vi "Check_Execution_Row.vi"(0 "Execution Row":T1 {"Row Duration (mins)" format="%#.1f"; "Row No" min=0; "Trace Gas Concentration (%)" min=0.0 format="%#.2f"; "Emission Rate (l/min)" format="%#.2f"; "Tunnel Speed" format="%#.2f"; "Start X" format="%#.2f"; "Start Y" format="%#.2f"; "Start Z" format="%#.2f"; "End X" format="%#.2f"; "End Y" format="%#.2f"; "End Z" format="%#.2f"; "Averaging time (min)" min=0.0 format="%#.2f"}, 3 "Synchronization Start No":i32=1 min=1 max=100, 4 "Row Index":i32, 5 "Max Tunnel Speed":dbl format="%.2f") -> (6 "Editted Row":bool, 7 "Execution Row Out":T1 {"Row Duration (mins)" format="%#.1f"; "Row No" min=0; "Trace Gas Concentration (%)" min=0.0 format="%#.2f"; "Emission Rate (l/min)" format="%#.2f"; "Tunnel Speed" format="%#.2f"; "Start X" format="%#.2f"; "Start Y" format="%#.2f"; "Start Z" format="%#.2f"; "End X" format="%#.2f"; "End Y" format="%#.2f"; "End Z" format="%#.2f"; "Averaging time (min)" min=0.0 format="%#.2f"}, 9 "Continue?":bool, 10 "Error Comments":string)   [LabVIEW 2011]
uses:
  Traverse_cluster.ctl
  Spacing.ctl
  Controls/Multi_run_mode.ctl
  Controls/User_Specific_mode.ctl
  Controls/Tunnel_Coordinates.ctl
  ADAM Client/Sub VIs/ADAM Controls/Channel_names.ctl
  Globals/Extra_Commands_Global.vi
  Globals/Constants_global.vi
  Globals/Trav_pos_global.vi
panel:
  out "Traverse line Out":T1 {"Row Duration (mins)" format="%#.1f"; "Row No" min=0; "Trace Gas Concentration (%)" min=0.0 format="%#.2f"; "Emission Rate (l/min)" format="%#.2f"; "Tunnel Speed" format="%#.2f"; "Start X" format="%#.2f"; "Start Y" format="%#.2f"; "Start Z" format="%#.2f"; "End X" format="%#.2f"; "End Y" format="%#.2f"; "End Z" format="%#.2f"; "Averaging time (min)" min=0.0 format="%#.2f"}
  out "Fixed Axis":bool[](array[boolean])
  out "Filenames":string[](array[string])
  out "Current Sync Number":i32
  out "Checks":string[](array[string])
  in  "Edit in Excel":bool
  in  "OK":bool
  # "X           Y            Z"
  # "Start"
  # "End"
  # "X           Y            Z"
  # "Start"
  # "End"
  # "X           Y            Z"
  # "Start"
  # "End"
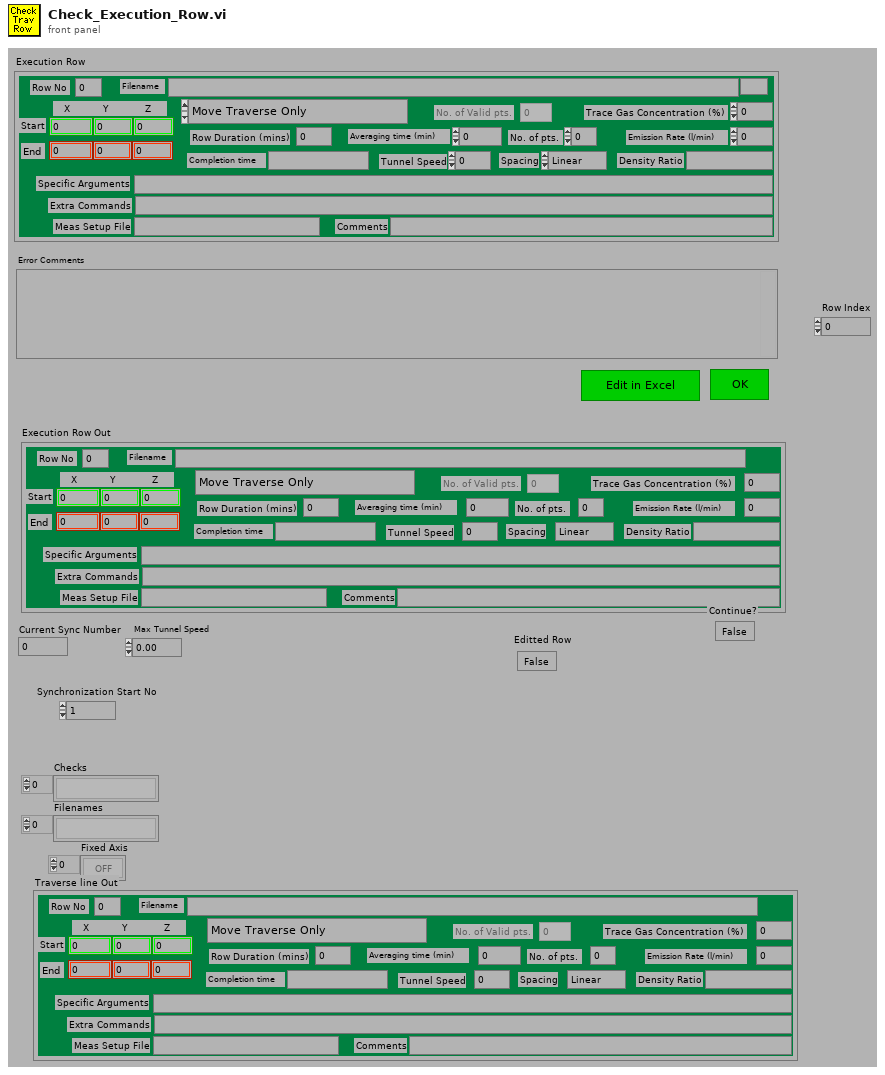
[diagram p1: front panel]
types:
  T1 = typedef "Traverse_cluster.ctl" = cluster{"Start X":dbl, "Start Y":dbl, "Start Z":dbl, "End X":dbl, "End Y":dbl, "End Z":dbl, "No. of pts.":i32, "Spacing":T2, "Filename":path, "Tunnel Speed":dbl, "Averaging time (min)":dbl, "Extra Commands":string, "Specific Arguments":string, "Emission Rate (l/min)":dbl, "Trace Gas Concentration (%)":dbl, "Density Ratio":string, "Comments":string, "Row No":i32, "Row Type Selector":T3, "Completion time":string, "Row Duration (mins)":dbl, "No. of Valid pts.":i32, "Meas Setup File":string}
  T2 = typedef "Spacing.ctl" = enum16{"Linear", "Log", "Gauss", "Specified", "N/A"}
  T3 = typedef "Multi_run_mode.ctl" = enum16{"Move Traverse Only", "Set Tunnel Speed Only", "Set Source Only", "Set Measurement Conditions", "Single Measurement", "Vertical Profile", "Lateral Profile", "Longitudinal Profile", "Explore Volume", "Multi-Axis Profile", "Auto Calibrate", "Meas Fast FID Bkgnd", "Check Beam Power", "Scanning Valve Measurement", "Run VI Named:", "Set ADAM Ch", "Wait (minutes)", "Send Message", "Synchronize With:", "Fall Back to this Row", "Turn Off Row Repeating", "Blank Row", "Traverse 3D Volume"}
  T4 = enum16{"All Channel Names", "Valid Channel Names"}
  T5 = typedef "User_Specific_mode.ctl" = enum16{"Check VI only", "Run VI"}
  T6 = typedef "Tunnel_Coordinates.ctl" = enum16{"Work in Tunnel Coordinates", "Work in Model Coordinates"}
  T7 = enum16{"Zero or one", "One", "Zero or more", "One or more"}
  T8 = typedef "Channel_names.ctl" = enum16{"Active Only", "Active + Off", "All Channels"}
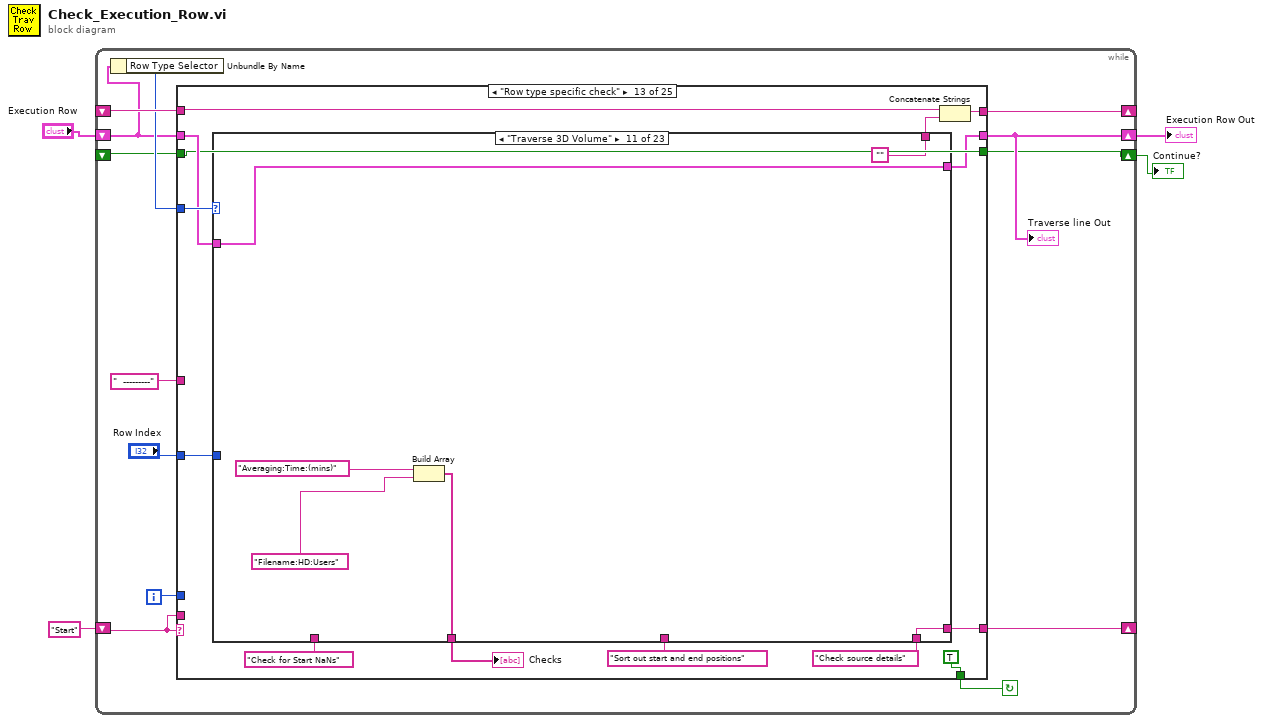
[diagram p0: block diagram]
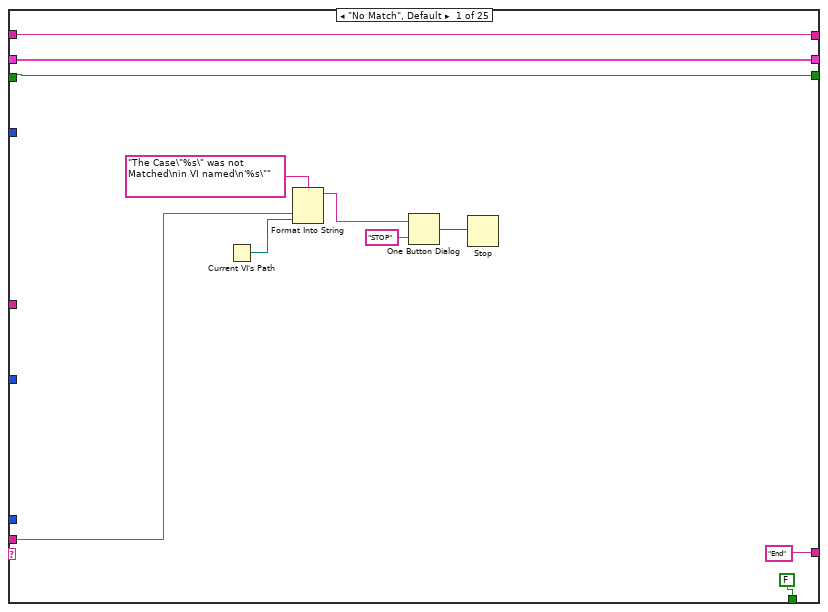
[diagram p2: hidden frame]
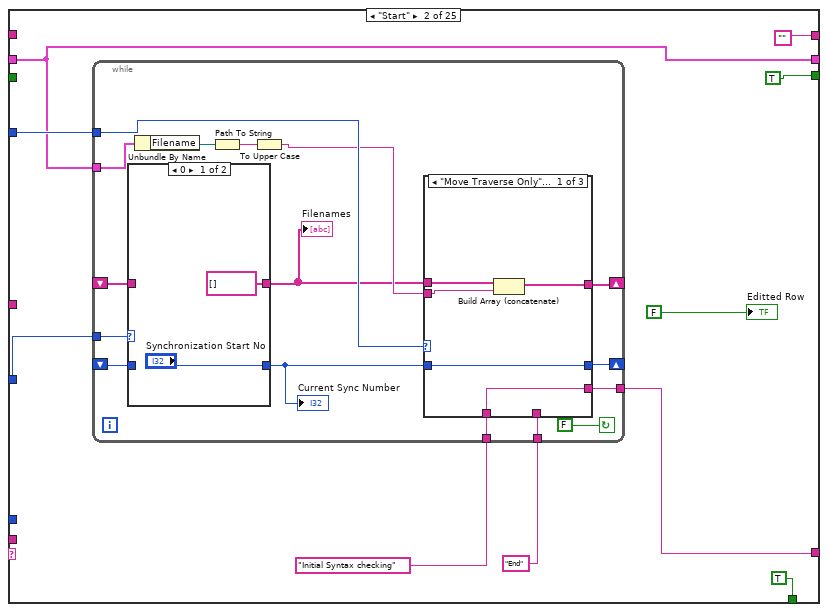
[diagram p3: hidden frame]
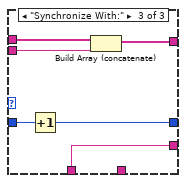
[diagram p6: hidden frame]
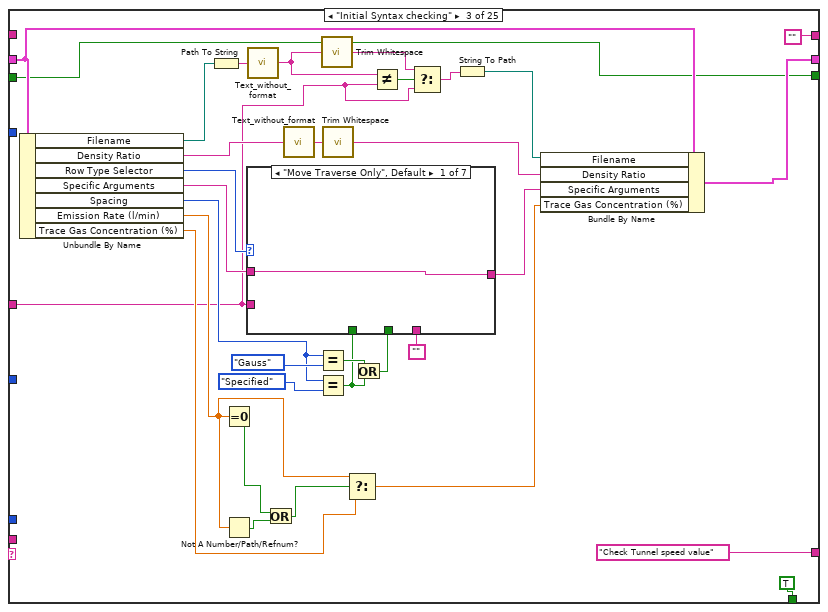
[diagram p7: hidden frame]
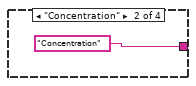
[diagram p9: hidden frame]
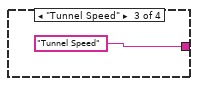
[diagram p10: hidden frame]
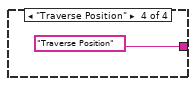
[diagram p11: hidden frame]
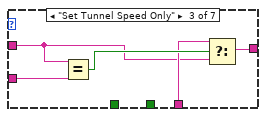
[diagram p12: hidden frame]
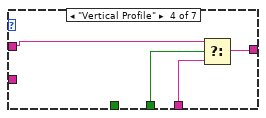
[diagram p13: hidden frame]
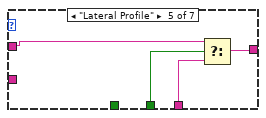
[diagram p14: hidden frame]
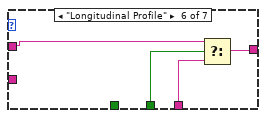
[diagram p15: hidden frame]
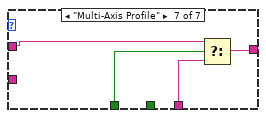
[diagram p16: hidden frame]
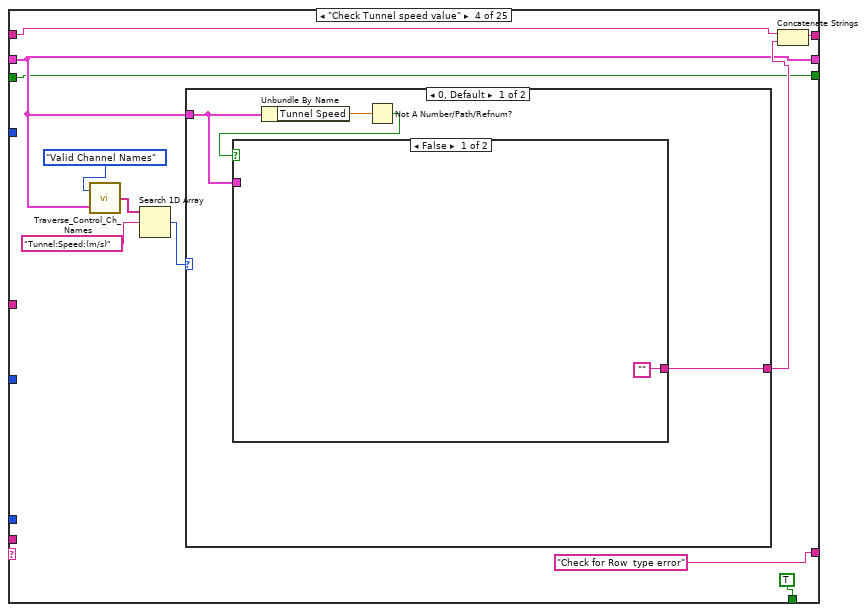
[diagram p17: hidden frame]
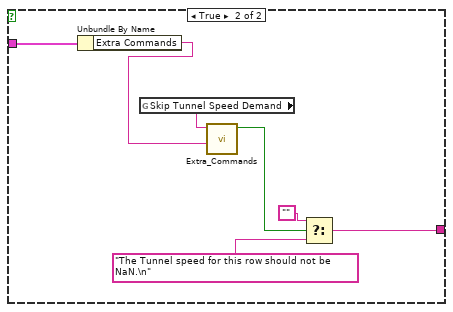
[diagram p18: hidden frame]
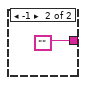
[diagram p19: hidden frame]
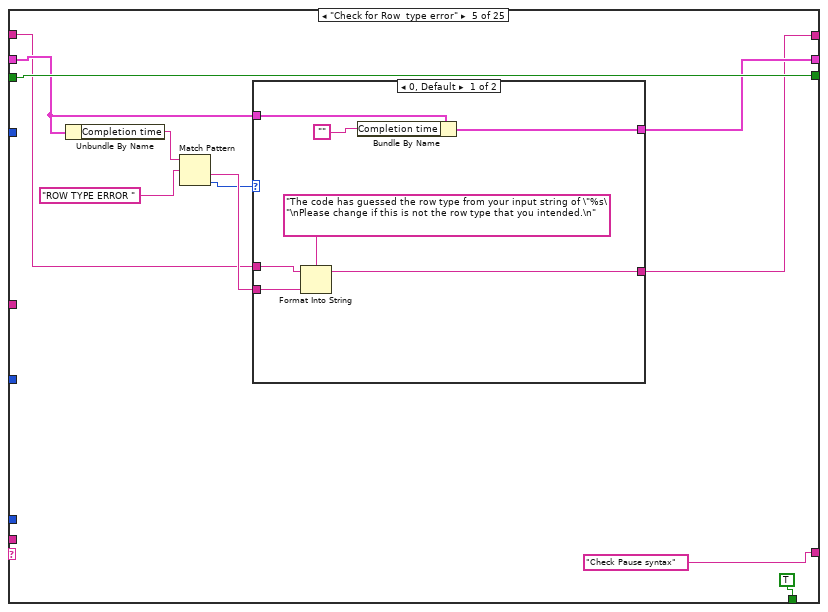
[diagram p20: hidden frame]
diagram:
  n1 = while {
    shift-left: _ -> [w16]
    shift-right: [w17] -> _
    shift-left: "Start" -> [w9]
    shift-right: [w14] -> _
    shift-right: [w8] -> w2
    shift-left: "Execution Row" -> [w5]
    shift-right: [w7] -> w1
    shift-left: _ -> [w6]
    i -> [w10]
    stop <- w15 continue-if-true
    n2 = Unbundle By Name(w5) -> ("Row Type Selector"=w12:T3)
    n3 = case shown="\"Row type specific check\"" w9 {
      tunnel: w5 -> [w22 w32 w100 w137 w161 w191 w205 w248 w278 w334 w367 w375 w414 w751 w851 w888 w916 w1001 w1033 w1043 w1112 _ w1151 w1158 w1168]
      tunnel: "  ---------" ("f") -> [_ _ w74 _ _ w195 _ _ _ _ _ _ _ _ _ _ _ _ _ _ _ _ _ _ _]
      tunnel: "Row Index" -> [_ w36 _ _ _ _ w202 _ _ _ _ _ w408 _ _ _ _ _ _ _ _ _ w1152 _ w1167]
      tunnel: [w21 "" "" w138 w158 w183 w213 w253 w283 w336 w371 w380 w418 w756 w861 w894 w939 w999 w1037 w1044 w1118 w1129 w1153 w1163 w1170] -> w17
      tunnel: w12 -> [_ w35 _ _ _ _ _ _ _ _ _ w378 w417 w752 w849 _ _ _ _ w1048 _ _ _ _ _]
      tunnel: w16 -> [w21 _ _ w139 w159 w185 w214 w254 w284 w336 w370 w381 w419 w756 w862 w895 w940 w999 w1038 w1049 w1118 w1129 w1153 w1163 w1170]
      tunnel: [FALSE TRUE TRUE TRUE TRUE TRUE TRUE TRUE TRUE TRUE TRUE TRUE TRUE TRUE TRUE TRUE TRUE TRUE TRUE w1040 TRUE TRUE TRUE TRUE FALSE] -> w15
      tunnel: ["End" w33 "Check Tunnel speed value" ("f") "Check for Row  type error" ("f") "Check Pause syntax" ("f") w188 "Check Traverse Setup Name" ("f") "Check IF command" ("f") "Check Measurement Setup?" ("f") w338 "Check Maximum tunnel speed" ("f") "Row type specific check" ("f") w415 "Check for position NaNs" ("f") w852 "Check source details" ("t") "Check source details" ("f") w996 "check entered filename etc" ("f") w1046 "What to do next?" ("f") w1127 "Initial Syntax checking" "End" "End"] -> w14
      tunnel: w10 -> [_ _ _ _ _ _ _ _ _ _ _ _ _ _ _ _ _ _ _ _ _ _ _ _ _]
      tunnel: w9 -> [w23 _ _ _ _ _ _ _ _ _ _ _ _ _ _ _ _ _ _ _ _ _ _ _ _]
      tunnel: [w22 w32 w77 w137 w162 w178 w204 w248 w278 w334 w366 w375 w409 w750 w851 w888 w915 w1000 w1033 w1042 w1112 w1120 w1154 w1158 w1166] -> w8
      tunnel: [w18 TRUE w75 w136 w168 w179 w206 w245 w275 w340 w368 w373 w411 w748 w850 w887 w913 w1004 w1031 w1040 w1111 w1119 w1148 w1157 w1164] -> w7
      tunnel: w6 -> [w18 _ w75 w136 w168 w179 w206 w245 w275 w340 w368 w373 w411 w748 w850 w887 w913 w1004 w1031 _ w1111 _ w1148 w1157 w1164]
      frame "No Match", Default {
        n4 = Current VI's Path() -> (path=w24:path)
        n5 = Format Into String(format string="The Case\"%s\" was not Matched\nin VI named\n'%s\"" ("Format String"), w23, w24) -> (resulting string=w27:string)  [unwired: 2 in, 1 out]
        n6 = One Button Dialog(message=w27, button name ("OK")="STOP") -> (true=w25:bool)
        n7 = Stop(stop? (T)=w25) -> ()
      }
      frame "Start" {
        n8 = while {
          tunnel: "End" -> [w40]
          tunnel: "Initial Syntax checking" -> [w41]
          tunnel: [w42] -> w33
          tunnel: w32 -> [w49]
          shift-left: _ -> [w48]
          shift-right: [w47] -> _
          tunnel: w35 -> [w53]
          shift-left: _ -> [w52]
          shift-right: [w51] -> _
          tunnel: w36 -> [w54]
          stop <- FALSE continue-if-true
          n9 = case shown="0" w54 {
            tunnel: ["Synchronization Start No" w58] -> w50
            tunnel: w52 -> [_ w58]
            tunnel: w48 -> [_ w57]
            tunnel: [string[] [] w57] -> w43
            frame 0 {
            }
            frame 1, Default {
            }
          }
          "Current Sync Number" <- w50
          "Filenames" <- w43
          n10 = Unbundle By Name(w49) -> ("Filename"=w46:path)
          n11 = Path To String(path=w46) -> (string=w45:string)
          n12 = To Upper Case(1:w45) -> (0:w44:string)
          n13 = case shown="\"Move Traverse Only\", Default" w53 {
            tunnel: w50 -> [w63 w66 w72]
            tunnel: [w63 w66 w71] -> w51
            tunnel: w44 -> [w61 _ w70]
            tunnel: w43 -> [w62 w65 w69]
            tunnel: [w60 w65 w68] -> w47
            tunnel: [w59 w64 w67] -> w42
            tunnel: w41 -> [w59 _ w67]
            tunnel: w40 -> [_ w64 _]
            frame "Move Traverse Only", Default {
              n14 = Build Array (concatenate)(w62, w61) -> (w60:string[])
            }
            frame "Blank Row" {
            }
            frame "Synchronize With:" {
              n15 = Increment(x=w72) -> (x+1=w71:i32)
              n16 = Build Array (concatenate)(w69, w70) -> (w68:string[])
            }
          }
        }
        "Editted Row" <- FALSE ("Editted Row")
      }
      frame "Initial Syntax checking" {
        n17 = Unbundle By Name(w100) -> ("Filename"=w73:path, "Density Ratio"=w79:string, "Row Type Selector"=w97:T3, "Specific Arguments"=w95:string, "Spacing"=w87:T2, "Emission Rate (l/min)"=w83:dbl, "Trace Gas Concentration (%)"=w93:dbl)
        n18 = Path To String(path=w73) -> (string=w81:string)
        n19 = Equal To 0?(x=w83) -> (x = 0?=w85:bool)
        n20 = Not A Number/Path/Refnum?(number/path/refnum=w83) -> (NaN/Path/Refnum?=w84:bool)
        n21 = call "Text_without_format.vi"("Input string"=w81) -> ("Output string"=w104:string)
        n22 = Or(x=w85, y=w84) -> (x .or. y?=w82:bool)
        n23 = call "Text_without_format.vi"("Input string"=w79) -> ("Output string"=w99:string)
        n24 = Equal?(x=w87, y=Spacing."Gauss" ("Spacing")) -> (x = y?=w89:bool)
        n25 = Equal?(x=w87, y=Spacing."Specified" ("Spacing")) -> (x = y?=w86:bool)
        n26 = call <vilib>:"Trim Whitespace.vi"("string"=w104) -> ("trimmed string"=w103:string)  [unwired: 1 in]
        n27 = call <vilib>:"Trim Whitespace.vi"("string"=w99) -> ("trimmed string"=w78:string)  [unwired: 1 in]
        n28 = Select(t=w83, s=w82, f=w93) -> (s? t:f=w92:dbl)
        n29 = Or(x=w89, y=w86) -> (x .or. y?=w88:bool)
        n30 = case shown="\"Move Traverse Only\", Default" w97 {
          tunnel: [w106 w108 w113 w119 w123 w127 w131] -> w96
          tunnel: w95 -> [w106 w107 w114 w121 w125 w129 w133]
          tunnel: "" -> [_ _ w115 w120 w124 w128 w132]
          tunnel: w88 -> [_ _ _ w118 w122 w126 _]
          tunnel: w86 -> [_ _ _ _ _ _ w130]
          tunnel: w74 -> [_ _ w117 _ _ _ _]
          frame "Move Traverse Only", Default {
          }
          frame "Auto Calibrate" {
            n31 = case shown="\"No Match\", Default" w107 {
              tunnel: [w109 "Concentration" "Tunnel Speed" "Traverse Position"] -> w108
              tunnel: w107 -> [w109 _ _ _]
              frame "No Match", Default {
              }
              frame "Concentration" {
              }
              frame "Tunnel Speed" {
              }
              frame "Traverse Position" {
              }
            }
          }
          frame "Set Tunnel Speed Only" {
            n32 = Equal?(x=w114, y=w117) -> (x = y?=w116:bool)
            n33 = Select(t=w115, s=w116, f=w114) -> (s? t:f=w113:string)
          }
          frame "Vertical Profile" {
            n34 = Select(t=w121, s=w118, f=w120) -> (s? t:f=w119:string)
          }
          frame "Lateral Profile" {
            n35 = Select(t=w125, s=w122, f=w124) -> (s? t:f=w123:string)
          }
          frame "Longitudinal Profile" {
            n36 = Select(t=w129, s=w126, f=w128) -> (s? t:f=w127:string)
          }
          frame "Multi-Axis Profile" {
            n37 = Select(t=w133, s=w130, f=w132) -> (s? t:f=w131:string)
          }
        }
        n38 = Not Equal?(x=w104, y=w74) -> (x != y?=w105:bool)
        n39 = Select(t=w103, s=w105, f=w74) -> (s? t:f=w102:string)
        n40 = String To Path(string=w102) -> (path=w80:path)
        n41 = Bundle By Name(cluster=w100, "Filename"=w80, "Density Ratio"=w78, "Specific Arguments"=w96, "Trace Gas Concentration (%)"=w92) -> (w77:T1)
      }
      frame "Check Tunnel speed value" {
        n42 = call "Traverse_Control_Ch_Names.vi"("Traverse line"=w137, "Mode"=T4."Valid Channel Names") -> ("Channel names"=w143:string[])
        n43 = Search 1D Array(1D array=w143, element="Tunnel:Speed:(m/s)" ("Label for value")) -> (index of element=w141:i32)  [unwired: 1 out]
        n44 = case shown="0, Default" w141 {
          tunnel: w137 -> [w146 _]
          tunnel: [w145 ""] -> w140
          frame 0, Default {
            n45 = Unbundle By Name(w146) -> ("Tunnel Speed"=w148:dbl)
            n46 = Not A Number/Path/Refnum?(number/path/refnum=w148) -> (NaN/Path/Refnum?=w147:bool)
            n47 = case shown="False" w147 {
              tunnel: w146 -> [_ w156]
              tunnel: ["" w150] -> w145
              frame False {
              }
              frame True {
                n48 = Unbundle By Name(w156) -> ("Extra Commands"=w154:string)
                n49 = global read "Extra_Commands_Global.vi" "Skip Tunnel Speed Demand"() -> (w155:string)
                n50 = call "Extra_Commands.vi"("String to Search"=w154, "Command"=w155) -> ("Command Found"=w153:bool)  [unwired: 1 in, 4 out]
                n51 = Select(t="", s=w153, f="The Tunnel speed for this row should not be NaN.\n") -> (s? t:f=w150:string)
              }
            }
          }
          frame -1 {
          }
        }
        n52 = Concatenate Strings(w139, w140) -> (w138:string)
      }
      frame "Check for Row  type error" {
        n53 = Unbundle By Name(w161) -> ("Completion time"=w164:string)
        n54 = Match Pattern(string=w164, regular expression="ROW TYPE ERROR " ("format string")) -> (after substring=w163:string, offset past match=w160:i32)  [unwired: 3 out]
        n55 = case shown="0, Default" w160 {
          tunnel: w163 -> [w175 _]
          tunnel: [w173 w177] -> w162
          tunnel: w161 -> [w172 w177]
          tunnel: [w170 w176] -> w158
          tunnel: w159 -> [w169 w176]
          frame 0, Default {
            n56 = Format Into String(format string="The code has guessed the row type from your input string of \"%s\"\nPlease change if this is not the row type that you intended.\n", initial string=w169, w175) -> (resulting string=w170:string)  [unwired: 1 in, 1 out]
            n57 = Bundle By Name(cluster=w172, "Completion time"="") -> (w173:T1)
          }
          frame -1 {
          }
        }
      }
      frame "Check Pause syntax" {
        n58 = Unbundle By Name(w191) -> ("Extra Commands"=w196:string)
        n59 = Not Equal?(x=w196, y=w195) -> (x != y?=w197:bool)
        n60 = Select(t=w196, s=w197, f="") -> (s? t:f=w193:string)
        n61 = call <vilib>:"Trim Whitespace.vi"("string"=w193) -> ("trimmed string"=w187:string)  [unwired: 1 in]
        n62 = Equal?(x=w187, y="") -> (x = y?=w189:bool)
        n63 = call "Pause_for_server_ch_val.vi"("Extra command string"=w187, "Simulate/Run"=User_Specific_mode."Check VI only") -> ("Extra command string Out"=w186:string, "Error Comments"=w184:string)
        n64 = Bundle By Name(cluster=w191, "Extra Commands"=w186) -> (w178:T1)
        n65 = Concatenate Strings(w185, w184) -> (w183:string)
        n66 = Select(t="Check Measurement Setup?", s=w189, f="Check Extra Commands") -> (s? t:f=w188:string)
      }
      frame "Check Extra Commands" {
        n67 = Unbundle By Name(w205) -> ("Extra Commands"=w207:string)
        n68 = for {
          N: 4 -> [_]
          tunnel: w207 -> [w222]
          shift-right: [w218] -> w210
          shift-left: "" -> [w219]
          i -> [w224]
          n69 = case shown="0, Default" w224 {
            tunnel: [w227 w229 w231 w233] -> w221
            tunnel: ["The Extra Command \"%s\" should have a numeric argument.\n" ("Format String") "The Extra Command \"%s\" should have a numeric argument.\n" ("Format String") "The Extra Command \"%s\" should have a numeric argument.\n" ("Format String") "The Extra Command \"%s\" should have a numeric argument.\n" ("Format String")] -> w216
            frame 0, Default {
              n70 = global read "Extra_Commands_Global.vi" "Coil Analysis time (s)"() -> (w227:string)
            }
            frame 1 {
              n71 = global read "Extra_Commands_Global.vi" "Estimated Av Csample/Csource"() -> (w229:string)
            }
            frame 2 {
              n72 = global read "Extra_Commands_Global.vi" "Establish Exp Conditions (s)"() -> (w231:string)
            }
            frame 3 {
              n73 = global read "Extra_Commands_Global.vi" "Minutes Before Repeating Row"() -> (w233:string)
            }
          }
          n74 = call "Extra_Commands.vi"("String to Search"=w222, "Command"=w221) -> ("String Value"=w223:string, "Command Found"=w225:bool)  [unwired: 1 in, 3 out]
          n75 = case shown="False" w225 {
            tunnel: w223 -> [_ w242]
            tunnel: w221 -> [_ w240]
            tunnel: [w234 w237] -> w220
            tunnel: "" -> [w234 w236]
            tunnel: w216 -> [_ w235]
            frame False {
            }
            frame True {
              n76 = Decimal String To Number(string=w242) -> (offset past number=w241:i32)  [unwired: 3 out]
              n77 = Equal To 0?(x=w241) -> (x = 0?=w239:bool)
              n78 = Format Into String(format string=w235, w240) -> (resulting string=w238:string)  [unwired: 2 in, 1 out]
              n79 = Select(t=w238, s=w239, f=w236) -> (s? t:f=w237:string)
            }
          }
          n80 = Concatenate Strings(w220, w219) -> (w218:string)
        }
        n81 = call "Trav_Prog_Extra_Commands.vi"() -> ("Extra Commands Array"=w208:string[])  [unwired: 2 out]
        n82 = call "Valid_Extra_Command.vi"("Extra Commands string"=w207, "Valid Commands Array"=w208) -> ("Output String"=w212:string, "Extra Commands string Out"=w203:string)  [unwired: 3 out]
        n83 = Bundle By Name(cluster=w205, "Extra Commands"=w203) -> (w204:T1)
        n84 = call "Skip_If Sd_Error_Below.vi"("String to Search"=w203, "Simulate/Run"=User_Specific_mode."Check VI only", "Measurement setup Applied?"=FALSE, "Row Number"=w202) -> ("Error String"=w199:string)  [unwired: 1 in, 4 out]
        n85 = Concatenate Strings(w214, w212, w210, w199) -> (w213:string)
      }
      frame "Check Traverse Setup Name" {
        n86 = Unbundle By Name(w248) -> ("Extra Commands"=w244:string)
        n87 = global read "Extra_Commands_Global.vi" "!Traverse Setup"() -> (w251:string)
        n88 = call "Extra_Commands.vi"("String to Search"=w244, "Command"=w251) -> ("String Value"=w249:string, "Command Found"=w250:bool)  [unwired: 1 in, 3 out]
        n89 = case shown="True" w250 {
          tunnel: w249 -> [_ w261]
          tunnel: [w255 w258] -> w246
          tunnel: "" -> [w255 w257]
          frame False {
          }
          frame True {
            n90 = global read "Constants_global.vi" "Traverse folder"() -> (w256:path)
            n91 = List Folder(path=w256) -> (folder names=w259:string[])  [unwired: 1 in, 5 out]
            n92 = Search 1D Array(1D array=w259, element=w261) -> (index of element=w262:i32)  [unwired: 1 out]
            n93 = Greater Or Equal To 0?(x=w262) -> (x >= 0?=w260:bool)
            n94 = case shown="False" w260 {
              tunnel: w261 -> [w267 _]
              tunnel: w259 -> [w264 _]
              tunnel: [w263 w272] -> w258
              tunnel: w257 -> [_ w272]
              frame False {
                n95 = Format Into String(format string="%s is not a valid Travese setup. Valid option are:", w267) -> (resulting string=w265:string)  [unwired: 2 in, 1 out]
                n96 = for {
                  shift-right: [w269] -> w263
                  shift-left: w265 -> [w270]
                  tunnel: w264 -> [w271] mode=indexing
                  w268 = "  " ("Substring")
                  n97 = Concatenate Strings(w270, w268, w271, w268) -> (w269:string)
                }
              }
              frame True {
              }
            }
          }
        }
        n98 = Concatenate Strings(w254, w246) -> (w253:string)
      }
      frame "Check IF command" {
        n99 = Unbundle By Name(w278) -> ("Extra Commands"=w274:string)
        n100 = global read "Extra_Commands_Global.vi" "If Command"() -> (w281:string)
        n101 = call "Extra_Commands.vi"("String to Search"=w274, "Command"=w281) -> ("String Value"=w279:string, "Command Found"=w280:bool)  [unwired: 1 in, 3 out]
        n102 = case shown="True" w280 {
          tunnel: w279 -> [_ w290]
          tunnel: [w285 w289] -> w276
          tunnel: "" -> [w285 w287]
          frame False {
          }
          frame True {
            n103 = call "Get_array_values_fr_String.vi"("String Value"=w290) -> ("Numeric Array"=w286:dbl[], "String array"=w288:string[])
            n104 = Index Array(array=w288, index=0 ("Index")) -> (element=w291:string)
            n105 = case shown="\"Global Value Between\"" w291 {
              tunnel: w290 -> [w296 _ _ _]
              tunnel: [w295 w321 w322 "The !If  command has not been recognised.\nExtra command Example:\n!IF = Time Between;10:45;and;14:00;Execute Row (or) Skip Row\n\n!IF = ADAM Channel Between;Channel Name; 0.5;1.0\n\n!IF = Global Value Between; 0.5;1.0" ("Error Comments")] -> w289
              tunnel: w288 -> [_ w312 w330 _]
              tunnel: w287 -> [_ w305 w323 _]
              tunnel: w286 -> [_ _ _ _]
              frame "Time Between" {
                n106 = Get Date/Time In Seconds() -> (seconds since 1Jan1904=w293:timestamp)
                n107 = To Double Precision Float(number=w293) -> (double precision float=w294:dbl)
                n108 = call "If_Time_arguments.vi"("seconds since 1Jan1904"=w294, "String Value"=w296) -> ("Error Comments"=w295:string)  [unwired: 2 out]
              }
              frame "ADAM Channel Between" {
                n109 = Index Array(array=w312, index=1 ("Index")) -> (element=w315:string)
                n110 = Index Array(array=w312, index=2 ("Index")) -> (element=w311:string)
                n111 = Index Array(array=w312, index=3 ("Index")) -> (element=w310:string)
                n112 = Build Array(w315) -> (w317:string[])
                n113 = Decimal Digit?(1:w311) -> (0:w308:bool)
                n114 = Decimal Digit?(1:w310) -> (0:w309:bool)
                n115 = call "Get_Current_Scan_client.vi"("ADAM Ch Names"=w317) -> ("Numerical Values"=w319:dbl[])  [unwired: 3 out]
                n116 = And(x=w308, y=w309) -> (x .and. y?=w307:bool)
                n117 = Index Array(array=w319, index=0 ("Index")) -> (element=w320:dbl)
                n118 = Select(t=w305, s=w307, f="you must give two limits\n") -> (s? t:f=w301:string)
                n119 = Not A Number/Path/Refnum?(number/path/refnum=w320) -> (NaN/Path/Refnum?=w304:bool)
                n120 = Select(t="Invalid ADAM Channel Name\n", s=w304, f=w305) -> (s? t:f=w302:string)
                n121 = Concatenate Strings(w302, w301) -> (w299:string)
                n122 = Concatenate Strings(w299, "Extra command Example:\n!IF = ADAM Channel Between;Channel Name; 0.5;1.0") -> (w298:string)
                n123 = Empty String/Path?(string/path=w299) -> (empty?=w300:bool)
                n124 = Select(t=w305, s=w300, f=w298) -> (s? t:f=w321:string)
              }
              frame "Global Value Between" {
                n125 = Index Array(array=w330, index=1 ("Index")) -> (element=w329:string)
                n126 = Index Array(array=w330, index=2 ("Index")) -> (element=w328:string)
                n127 = Decimal Digit?(1:w329) -> (0:w326:bool)
                n128 = Decimal Digit?(1:w328) -> (0:w327:bool)
                n129 = And(x=w326, y=w327) -> (x .and. y?=w325:bool)
                n130 = Select(t=w323, s=w325, f="The Extra command IF statement must have two numerical values for the limits\n\nExtra command Example:\n!IF = Global Value Between; 0.5;1.0") -> (s? t:f=w322:string)
              }
              frame "No Match", Default {
              }
            }
          }
        }
        n131 = Concatenate Strings(w284, w276) -> (w283:string)
      }
      frame "Check Measurement Setup?" {
        n132 = Unbundle By Name(w334) -> ("Row Type Selector"=w339:T3, "Specific Arguments"=w337:string)
        n133 = case shown="\"Traverse 3D Volume\"" w339 {
          tunnel: ["Check Measurement Setup" ("t") "Check Measurement Setup" ("t") "Check Measurement Setup" ("t") "Check Measurement Setup" ("t") "Check Measurement Setup" ("t") "Check Measurement Setup" ("t") "Check Measurement Setup" ("t") "Check Measurement Setup" ("t") "Check Measurement Setup" ("t") "Check Measurement Setup" ("t") "Check Measurement Setup" ("t") w353 w362] -> w338
          tunnel: w337 -> [_ _ _ _ _ _ _ _ _ _ _ w360 _]
          tunnel: "Check Maximum tunnel speed" ("f") -> [_ _ _ _ _ _ _ _ _ _ _ w354 w362]
          tunnel: w334 -> [_ _ _ _ _ _ _ _ _ _ _ w357 _]
          frame "Lateral Profile" {
          }
          frame "Traverse 3D Volume" {
          }
          frame "Longitudinal Profile" {
          }
          frame "Explore Volume" {
          }
          frame "Multi-Axis Profile" {
          }
          frame "Vertical Profile" {
          }
          frame "Single Measurement" {
          }
          frame "Scanning Valve Measurement" {
          }
          frame "Auto Calibrate" {
          }
          frame "Meas Fast FID Bkgnd" {
          }
          frame "Check Beam Power" {
          }
          frame "Run VI Named:" {
            n134 = Match Pattern(string=w360, regular expression=";") -> (before substring=w359:string)  [unwired: 4 out]
            n135 = call <vilib>:"Trim Whitespace.vi"("string"=w359) -> ("trimmed string"=w358:string)  [unwired: 1 in]
            n136 = call "Run_VI_Named_specific.vi"("Run VI Named String"=w358, "Multi Run Row"=w357) -> ("Check Meas Setup?"=w356:bool)  [unwired: 9 out]
            n137 = Select(t="Check Measurement Setup", s=w356, f=w354) -> (s? t:f=w353:string)
          }
          frame "Set Tunnel Speed Only", Default {
          }
        }
      }
      frame "Check Measurement Setup" {
        n138 = Unbundle By Name(w367) -> ("Meas Setup File"=w365:string)
        n139 = call "Check_Measurement_Setups.vi"("Measurement Setup String"=w365) -> ("Measurement Setup String Out"=w364:string, "Error Comments"=w363:string)
        n140 = Bundle By Name(cluster=w367, "Meas Setup File"=w364) -> (w366:T1)
        n141 = Concatenate Strings(w370, w363) -> (w371:string)
      }
      frame "Check Maximum tunnel speed" {
        n142 = case shown="\"Set Tunnel Speed Only\", Default" w378 {
          tunnel: w375 -> [w400 _]
          tunnel: [w391 FALSE] -> w377
          tunnel: [w390 0.0] -> w376
          frame "Auto Calibrate" {
            n143 = Unbundle By Name(w400) -> ("Specific Arguments"=w399:string)
            n144 = call "Get_array_values_fr_String.vi"("String Value"=w399) -> ("Numeric Array"=w393:dbl[], "String array"=w398:string[])
            n145 = Index Array(array=w398, index=0 ("Index")) -> (element=w396:string)
            n146 = Equal?(x=w396, y="Tunnel Speed" ("Output Array")) -> (x = y?=w391:bool)
            n147 = Array Subset(array=w393, index=1 ("Array Index")) -> (w392:dbl[])  [unwired: 1 in]
            n148 = Array Max & Min(array=w392) -> (max value=w390:dbl)  [unwired: 3 out]
          }
          frame "Set Tunnel Speed Only", Default {
          }
        }
        n149 = case shown="False" w377 {
          tunnel: [w388 w389] -> w385
          tunnel: w375 -> [w387 _]
          tunnel: w376 -> [_ w389]
          frame False {
            n150 = Unbundle By Name(w387) -> ("Tunnel Speed"=w388:dbl)
          }
          frame True {
          }
        }
        n151 = Greater?(x=w385, y="Max Tunnel Speed") -> (0:w383:bool)
        n152 = Not A Number/Path/Refnum?(number/path/refnum=w385) -> (NaN/Path/Refnum?=w384:bool)
        n153 = Compound Arithmetic op=AND(invert w384, w383) -> (w382:bool)
        n154 = case shown="False" w382 {
          tunnel: w381 -> [w403 w405]
          tunnel: [w403 w404] -> w380
          tunnel: "Max Tunnel Speed" -> [_ w407]
          frame False {
          }
          frame True {
            n155 = Format Into String(format string="The maximum allowable tunnel speed is %.2f m/s.\n" ("Format String"), initial string=w405, w407) -> (resulting string=w404:string)  [unwired: 1 in, 1 out]
          }
        }
      }
      frame "Row type specific check" {
        n156 = case shown="\"Traverse 3D Volume\"" w417 {
          tunnel: w414 -> [w428 w437 w441 w445 w450 w455 w462 w469 w480 w488 w502 w520 w574 w581 w602 w630 w679 w707 w712 w716 w728 w732 w738]
          tunnel: [string[] [] string[] [] string[] [] string[] [] w451 w458 w465 w472 w485 w493 w503 w528 w576 string[] [] w619 string[] [] w674 string[] [] string[] [] string[] [] string[] [] string[] [] string[] []] -> w416
          tunnel: [w422 "" "" "" "" "" "" "" w481 w490 "" w542 w570 w580 w614 w622 w690 w709 "" w718 "" "" w740] -> w420
          tunnel: [w431 w438 w442 w446 w449 w456 w463 w470 w479 w489 w501 w527 w564 w579 w613 w633 w675 "check entered filename etc" "check entered filename etc" "check entered filename etc" "check entered filename etc" "check entered filename etc" "check entered filename etc"] -> w415
          tunnel: "Check source details" -> [_ w438 w442 _ _ _ _ _ _ _ w501 _ w564 w579 w613 w632 w676 _ _ _ _ _ _]
          tunnel: "Sort out start and end positions" -> [_ _ _ _ _ w456 w463 w470 _ w489 _ w525 _ _ _ _ _ _ _ _ _ _ _]
          tunnel: "Check for Start NaNs" -> [w431 _ _ w446 w449 _ _ _ w479 _ _ w526 _ _ _ _ _ _ _ _ _ _ _]
          tunnel: [w427 w437 w441 w445 w450 w455 w462 w469 w480 w488 w502 w506 w574 w589 w602 w629 w679 w707 w712 w716 w728 w732 w736] -> w409
          tunnel: w408 -> [_ _ _ _ _ _ _ _ _ _ _ _ _ _ _ w635 _ _ _ _ _ _ _]
          frame "Move Traverse Only" {
            n157 = Unbundle By Name(w428) -> ("Specific Arguments"=w429:string)
            n158 = call <vilib>:"Trim Whitespace.vi"("string"=w429) -> ("trimmed string"=w423:string)  [unwired: 1 in]
            n159 = Equal?(x=w423, y="No Backlash") -> (x = y?=w426:bool)
            n160 = Empty String/Path?(string/path=w423) -> (empty?=w425:bool)
            n161 = Or(x=w425, y=w426) -> (x .or. y?=w424:bool)
            n162 = case shown="True" w424 {
              tunnel: w423 -> [w434 _]
              tunnel: [w433 ""] -> w422
              frame False {
                n163 = Format Into String(format string="\"%s\" is an Incorrect Specific Argument. It should either be left blank or say \"No Backlash\"\n", w434) -> (resulting string=w433:string)  [unwired: 2 in, 1 out]
              }
              frame True {
              }
            }
            n164 = Bundle By Name(cluster=w428, "Specific Arguments"=w423) -> (w427:T1)
          }
          frame "Set Tunnel Speed Only" {
          }
          frame "Set Source Only" {
          }
          frame "Set Measurement Conditions" {
          }
          frame "Single Measurement" {
            n165 = Build Array("Averaging:Time:(mins)" ("Label for value"), "Filename:HD:Users" ("Label for value")) -> (w451:string[])
          }
          frame "Vertical Profile" {
            n166 = Build Array("Number:Of:Points" ("Label for value"), "Averaging:Time:(mins)" ("Label for value"), "Filename:HD:Users" ("Label for value")) -> (w458:string[])
          }
          frame "Lateral Profile" {
            n167 = Build Array("Number:Of:Points" ("Label for value"), "Averaging:Time:(mins)" ("Label for value"), "Filename:HD:Users" ("Label for value")) -> (w465:string[])
          }
          frame "Longitudinal Profile" {
            n168 = Build Array("Number:Of:Points" ("Label for value"), "Averaging:Time:(mins)" ("Label for value"), "Filename:HD:Users" ("Label for value")) -> (w472:string[])
          }
          frame "Explore Volume" {
            n169 = Unbundle By Name(w480) -> ("Specific Arguments"=w478:string)
            n170 = Build Array("Averaging:Time:(mins)" ("Label for value"), "Filename:HD:Users" ("Label for value")) -> (w485:string[])
            n171 = Fract/Exp String To Number(string=w478) -> (number=w477:dbl)  [unwired: 4 out]
            n172 = Greater Than 0?(x=w477) -> (x > 0?=w476:bool)
            n173 = Format Into String(format string="\"%s\" is an Incorrect Specific Argument. Please enter the radius of the volume in mm.\n", w478) -> (resulting string=w482:string)  [unwired: 2 in, 1 out]
            n174 = Select(t="", s=w476, f=w482) -> (s? t:f=w481:string)
          }
          frame "Multi-Axis Profile" {
            n175 = Unbundle By Name(w488) -> ("Spacing"=w491:T2)
            n176 = case shown="\"Gauss\"" w491 {
              tunnel: ["" "You are not allowed to specify gaussian spacing for a Multi-Axis profile.\n" "You are not allowed to specify Log spacing for a Multi-Axis profile.\n" "\"N/A\" is not a valid point spacing.\n"] -> w490
              frame "Linear", Default {
              }
              frame "Gauss" {
              }
              frame "Log" {
              }
              frame "N/A" {
              }
            }
            n177 = Build Array("Number:Of:Points" ("Label for value"), "Averaging:Time:(mins)" ("Label for value"), "Filename:HD:Users" ("Label for value")) -> (w493:string[])
          }
          frame "Traverse 3D Volume" {
            n178 = Build Array("Averaging:Time:(mins)" ("Label for value"), "Filename:HD:Users" ("Label for value")) -> (w503:string[])
          }
          frame "Auto Calibrate" {
            n179 = Unbundle By Name(w520) -> ("Filename"=w509:path, "Specific Arguments"=w541:string)
            n180 = call "Get_array_values_fr_String.vi"("String Value"=w541) -> ("Numeric Array"=w537:dbl[], "String array"=w524:string[])
            n181 = global read "Trav_pos_global.vi" "Work in Tunnel Coordinates?"() -> (w519:T6)
            n182 = Index Array(array=w524, index=0 ("Index")) -> (element=w523:string)
            n183 = Build Array("Tunnel Speed", "Traverse Position", "Concentration") -> (w522:string[])
            n184 = Build Array("Averaging:Time:(mins)" ("Label for value")) -> (w528:string[])
            n185 = Array Size(array=w537) -> (size(s)=w536:i32)
            n186 = call "Current_Filepath.vi"("Filename in"=w509, "Data Type"="Calibrations") -> ("Filename Out"=w507:path)  [unwired: 1 out]
            n187 = Equal?(x=w519, y=Tunnel_Coordinates."Work in Model Coordinates" ("Work in Tunnel Coordinates?")) -> (x = y?=w513:bool)
            n188 = Search 1D Array(1D array=w522, element=w523) -> (index of element=w514:i32)  [unwired: 1 out]
            n189 = Equal?(x=2, y=w514) -> (x = y?=w516:bool)
            n190 = case shown="1" w514 {
              tunnel: [w562 w563] -> w527
              tunnel: w526 -> [w562 _]
              tunnel: w525 -> [_ w563]
              frame 0, Default {
              }
              frame 1 {
              }
            }
            n191 = Less?(x=w536, y=3) -> (x < y?=w532:bool)
            n192 = Equal To 0?(x=w514) -> (x = 0?=w533:bool)
            n193 = And(x=w513, y=w516) -> (x .and. y?=w515:bool)
            n194 = Greater Or Equal To 0?(x=w514) -> (x >= 0?=w512:bool)
            n195 = Compound Arithmetic op=AND(w532, w533) -> (w531:bool)
            n196 = case shown="True" w515 {
              tunnel: w520 -> [w558 w560]
              tunnel: [w558 w559] -> w508
              frame False {
              }
              frame True {
                n197 = Bundle By Name(cluster=w560, "Comments"="WARNING POSITION IN TUNNEL COORDINATES!!") -> (w559:T1)
              }
            }
            n198 = Select(t="You need to enter the desired tunnel speeds in the \"Specfic Arguments\" Box   eg.  Tunnel Speed;1;2;3;4\n", s=w531, f="") -> (s? t:f=w529:string)
            n199 = call "Does_file_exist_(simple).vi"("Pathname"=w507) -> ("exists?"=w547:bool)
            n200 = case shown="False" w512 {
              tunnel: w522 -> [w549 _]
              tunnel: [w548 ""] -> w511
              frame False {
                n201 = for {
                  shift-right: [w554] -> w551
                  shift-left: "Incorrect Specific Argument. The options are: " -> [w555]
                  tunnel: w549 -> [w556] mode=indexing
                  w553 = "  " ("Substring")
                  n202 = Concatenate Strings(w555, w553, w556, w553) -> (w554:string)
                }
                n203 = Concatenate Strings(w551, "\r\n") -> (w548:string)
              }
              frame True {
              }
            }
            n204 = Select(t="", s=w547, f="The calibration file cannot be found.\n") -> (s? t:f=w543:string)
            n205 = Bundle By Name(cluster=w508, "Filename"=w507) -> (w506:T1)
            n206 = Concatenate Strings(w543, w529, w511) -> (w542:string)
          }
          frame "Meas Fast FID Bkgnd" {
            n207 = Unbundle By Name(w574) -> ("Specific Arguments"=w569:string)
            n208 = call "Get_array_values_fr_String.vi"("String Value"=w569) -> ("String array"=w568:string[])  [unwired: 1 out]
            n209 = Index Array(array=w568, index=0) -> (element=w566:string)
            n210 = Empty String/Path?(string/path=w566) -> (empty?=w572:bool)
            n211 = Build Array("Averaging:Time:(mins)" ("Label for value")) -> (w576:string[])
            n212 = Equal?(x=w566, y="Use Source Divertor Valve") -> (x = y?=w565:bool)
            n213 = Or(x=w572, y=w565) -> (x .or. y?=w571:bool)
            n214 = case shown="False" w571 {
              tunnel: ["Specific Argument should either be blank or\nUse Source Divertor Valve ; (wait time in seconds optional)" ""] -> w570
              frame False {
              }
              frame True {
              }
            }
          }
          frame "Check Beam Power" {
            n215 = Unbundle By Name(w581) -> ("Extra Commands"=w583:string, "Start X"=w588:dbl, "Start Y"=w586:dbl, "Start Z"=w587:dbl)
            n216 = global read "Extra_Commands_Global.vi" "Skip Traverse Position Demand"() -> (w584:string)
            n217 = call "Extra_Commands.vi"("String to Search"=w583, "Command"=w584) -> ("Command Found"=w582:bool)  [unwired: 1 in, 4 out]
            n218 = case shown="False" w582 {
              tunnel: w588 -> [w600 _]
              tunnel: w587 -> [w599 _]
              tunnel: w586 -> [w598 _]
              tunnel: "" -> [w595 w601]
              tunnel: [w594 w601] -> w580
              frame False {
                n219 = Build Array(w600, w598, w599) -> (w597:dbl[])
                n220 = Not A Number/Path/Refnum?(number/path/refnum=w597) -> (NaN/Path/Refnum?=w596:bool[])
                n221 = Or Array Elements(Boolean array=w596) -> (logical OR=w593:bool)
                n222 = Select(t="The start position is where the datum velocity measurement will be made. This should not contain NaNs.\n" ("f"), s=w593, f=w595) -> (s? t:f=w594:string)
              }
              frame True {
              }
            }
            n223 = Bundle By Name(cluster=w581, "Comments"="Start Position is the location of Datum Velocity Measurement") -> (w589:T1)
          }
          frame "Scanning Valve Measurement" {
            w615 = ext -0.5  # lo
            w616 = ext 47.5  # hi
            n224 = Unbundle By Name(w602) -> ("Specific Arguments"=w612:string)
            n225 = call "Get_array_values_fr_String.vi"("String Value"=w612) -> ("Numeric Array"=w611:dbl[], "String array"=w607:string[])
            n226 = Build Array("Averaging:Time:(mins)" ("Label for value"), "Filename:HD:Users" ("Label for value")) -> (w619:string[])
            n227 = Index Array(array=w607, index=0) -> (element=w606:string)
            n228 = Empty String/Path?(string/path=w606) -> (empty?=w604:bool)
            n229 = Index Array(array=w611, index=0) -> (element=w609:dbl)
            n230 = In Range and Coerce(upper limit=w616, x=w609, lower limit=w615) -> (In Range?=w605:bool)  [unwired: 1 out]
            n231 = Compound Arithmetic op=AND(invert w604, w605) -> (w603:bool)
            n232 = Select(t="", s=w603, f="Enter the scanning valve port number between 0 and 47 in the specific arguments box.\n") -> (s? t:f=w614:string)
          }
          frame "Set ADAM Ch" {
            n233 = while {
              shift-right: [w669] -> w637
              shift-left: _ -> [w662]
              shift-right: [w668] -> _
              shift-left: _ -> [w667]
              tunnel: w635 -> [w668]
              stop <- TRUE stop-if-true
              n234 = Array Size(array=w662) -> (size(s)=w666:i32)
              n235 = Less?(x=w668, y=w667) -> (x < y?=w664:bool)
              n236 = Equal To 0?(x=w666) -> (x = 0?=w665:bool)
              n237 = Or(x=w665, y=w664) -> (x .or. y?=w663:bool)
              n238 = case shown="True" w663 {
                tunnel: [w670 w671] -> w669
                tunnel: w662 -> [w670 _]
                frame False {
                }
                frame True {
                  n239 = call "Get_ADAM_Ch_names_client.vi"("Channel names set"=Channel_names."Active + Off") -> ("Ch names"=w671:string[])
                }
              }
            }
            n240 = Unbundle By Name(w630) -> ("Specific Arguments"=w641:string)
            n241 = call "Get_array_values_fr_String.vi"("String Value"=w641) -> ("String array"=w627:string[])  [unwired: 1 out]
            n242 = Index Array(array=w627, index=0) -> (element=w636:string)
            n243 = Search 1D Array(1D array=w637, element=w636) -> (index of element=w639:i32)  [unwired: 1 out]
            n244 = Index Array(array=w627, index=1) -> (element=w626:string)
            n245 = Empty String/Path?(string/path=w626) -> (empty?=w624:bool)
            n246 = Greater Or Equal To 0?(x=w639) -> (x >= 0?=w638:bool)
            n247 = Select(t="You have not specified a Value to Set the ADAM channel to.\nExample Specifice Argument:  ADAM_Ch_NAME  ;  10", s=w624, f="") -> (s? t:f=w622:string)
            n248 = case shown="False" w638 {
              tunnel: w637 -> [w658 _]
              tunnel: w636 -> [w656 _]
              tunnel: w635 -> [w654 _]
              tunnel: [w652 FALSE ("Cancel")] -> w634
              tunnel: w630 -> [w646 w659]
              tunnel: [w645 w659] -> w629
              tunnel: w626 -> [w643 _]
              frame False {
                n249 = Build Array(w656) -> (w655:string[])
                n250 = Format Into String(format string="Please Select the ADAM Channel that you want to set in row %d", w654) -> (resulting string=w653:string)  [unwired: 2 in, 1 out]
                n251 = call "Select_Strings.vi"("Available Ch names"=w658, "Message"=w653, "Selector mode"=T7."One", "Desired Ch names (in)"=w655) -> ("Cancel"=w652:bool, "Selected Channel Names"=w650:string[])  [unwired: 3 out]
                n252 = Index Array(array=w650, index=0) -> (element=w648:string)
                n253 = Concatenate Strings(w648, "  ;  " ("string"), w643) -> (w644:string)
                n254 = Bundle By Name(cluster=w646, "Specific Arguments"=w644) -> (w645:T1)
              }
              frame True {
              }
            }
            n255 = Select(t="Close Front Panel", s=w634, f=w632) -> (s? t:f=w633:string)
          }
          frame "Run VI Named:" {
            w684 = "Run_VI_Named_specific.vi"
            n256 = Unbundle By Name(w679) -> ("Specific Arguments"=w687:string)
            n257 = global read "Constants_global.vi" "Run VI Folder"() -> (w685:path)
            n258 = Match Pattern(string=w687, regular expression=";") -> (before substring=w688:string)  [unwired: 4 out]
            n259 = call <vilib>:"Trim Whitespace.vi"("string"=w688) -> ("trimmed string"=w680:string)  [unwired: 1 in]
            n260 = call "Run_VI_Named_specific.vi"("Run VI Named String"=w680, "Multi Run Row"=w679) -> ("Checks"=w674:string[], "Error String"=w673:string, "Check for start NaNs?"=w678:bool)  [unwired: 7 out]
            n261 = Select(t="Check for Start NaNs" ("Label for value"), s=w678, f=w676) -> (s? t:f=w675:string)
            n262 = Build Path(base path=w685, name or relative path=w680) -> (appended path=w691:path)
            n263 = Not Equal?(x=w680, y=w684) -> (x != y?=w683:bool)
            n264 = call "Does_file_exist_(simple).vi"("Pathname"=w691) -> ("exists?"=w682:bool)
            n265 = And(x=w682, y=w683) -> (x .and. y?=w681:bool)
            n266 = case shown="False" w681 {
              tunnel: [w698 ""] -> w686
              tunnel: w685 -> [w694 _]
              tunnel: w684 -> [w692 _]
              frame False {
                w696 = "\r\n"
                n267 = Build Array(w692) -> (w693:string[])
                n268 = call "List_files_in_order_of_age.vi"("Files to Hide"=w693, "Folder"=w694) -> ("file names"=w695:string[])
                n269 = for {
                  shift-right: [w702] -> w699
                  shift-left: "Cannot find the VI to run. Specific Argument options are:" -> [w703]
                  tunnel: w695 -> [w704] mode=indexing
                  w701 = "  " ("Substring")
                  n270 = Concatenate Strings(w703, w701, w704, w701) -> (w702:string)
                }
                n271 = Concatenate Strings(w699, w696, "Please place one of these strings in the \"Specific Argument\" field.", w696) -> (w698:string)
              }
              frame True {
              }
            }
            n272 = Concatenate Strings(w673, w686) -> (w690:string)
          }
          frame "Wait (minutes)" {
            n273 = Unbundle By Name(w707) -> ("Specific Arguments"=w708:string)
            n274 = call "Wait_Case_Arg.vi"("Specific Argument"=w708) -> ("Error Comments"=w709:string)  [unwired: 1 in, 4 out]
          }
          frame "Send Message" {
          }
          frame "Synchronize With:" {
            n275 = local read "Current Sync Number"() -> (w717:i32)
            n276 = call "Synchronize_Prog_Arg.vi"("Execution Row"=w716) -> ("Error Comments"=w719:string, "Sync No"=w725:i32)  [unwired: 3 out]
            n277 = Equal?(x=w725, y=w717) -> (x = y?=w724:bool)
            n278 = Format Into String(format string="This should be Synchroisation number %d.\n" ("Format String"), w717) -> (resulting string=w722:string)  [unwired: 2 in, 1 out]
            n279 = Select(t="", s=w724, f=w722) -> (s? t:f=w720:string)
            n280 = Concatenate Strings(w720, w719) -> (w718:string)
          }
          frame "Fall Back to this Row" {
          }
          frame "Turn Off Row Repeating" {
          }
          frame "Blank Row" {
            n281 = Unbundle By Name(w738) -> ("Comments"=w744:string)
            n282 = Match Pattern(string=w744, regular expression="(No Match Info)") -> (before substring=w737:string, after substring=w741:string)  [unwired: 3 out]
            n283 = Empty String/Path?(string/path=w741) -> (empty?=w742:bool)
            n284 = Bundle By Name(cluster=w738, "Comments"=w737) -> (w736:T1)
            n285 = Select(t=w741, s=w742, f="The Row Type Selector \"%s\" was not matched. Please select the desired type.\n") -> (s? t:f=w740:string)
          }
        }
        "Checks" <- w416
        n286 = Concatenate Strings(w419, w420) -> (w418:string)
      }
      frame "Sort out start and end positions" {
        n287 = Unbundle By Name(w751) -> ("Start X"=w763:dbl, "Start Y"=w762:dbl, "Start Z"=w761:dbl, "End X"=w760:dbl, "End Y"=w759:dbl, "End Z"=w758:dbl, "Extra Commands"=w747:string)
        n288 = call "Which_Trav_Setup.vi"("Extra Command String"=w747) -> ("Traverse Setup"=w746:string)
        n289 = call "Rig_Pict_Display_Pref.vi"("Traverse Name"=w746) -> ("Which Axis is vertical?"=w757:enum16{"X Axis", "Y Axis", "Z Axis"})  [unwired: 7 out]
        n290 = case shown="\"Multi-Axis Profile\", Default" w752 {
          tunnel: [w803 FALSE w819 w832 FALSE] -> w766
          tunnel: [w802 FALSE w818 w831 FALSE] -> w765
          tunnel: [w801 FALSE w817 w830 FALSE] -> w764
          tunnel: w757 -> [w800 _ w816 w829 _]
          frame "Vertical Profile" {
            n291 = case shown="\"Z Axis\"" w800 {
              tunnel: [FALSE TRUE TRUE] -> w803
              tunnel: [TRUE FALSE TRUE] -> w802
              tunnel: [TRUE TRUE FALSE] -> w801
              frame "X Axis" {
              }
              frame "Y Axis" {
              }
              frame "Z Axis" {
              }
            }
          }
          frame "Auto Calibrate" {
          }
          frame "Lateral Profile" {
            n292 = case shown="\"Y Axis\"" w816 {
              tunnel: [TRUE TRUE TRUE] -> w819
              tunnel: [TRUE TRUE FALSE] -> w818
              tunnel: [FALSE FALSE TRUE] -> w817
              frame "X Axis" {
              }
              frame "Y Axis" {
              }
              frame "Z Axis" {
              }
            }
          }
          frame "Longitudinal Profile" {
            n293 = case shown="\"Y Axis\"" w829 {
              tunnel: [FALSE FALSE FALSE] -> w832
              tunnel: [TRUE TRUE TRUE] -> w831
              tunnel: [TRUE TRUE TRUE] -> w830
              frame "X Axis" {
              }
              frame "Y Axis" {
              }
              frame "Z Axis" {
              }
            }
          }
          frame "Multi-Axis Profile", Default {
          }
        }
        n294 = Build Array(w763, w762, w761) -> (w754:dbl[])
        n295 = Build Array(w760, w759, w758) -> (w753:dbl[])
        n296 = Build Array(w766, w765, w764) -> (w755:bool[])
        "Fixed Axis" <- w755
        n297 = for {
          tunnel: w755 -> [w773] mode=indexing
          tunnel: w754 -> [w772] mode=indexing
          tunnel: w753 -> [w771] mode=indexing
          shift-right: [w768] -> w750
          shift-left: w751 -> [w769]
          i -> [w770]
          n298 = case shown="False" w773 {
            tunnel: w772 -> [_ w779]
            tunnel: w771 -> [_ w778]
            tunnel: w770 -> [_ w777]
            tunnel: w769 -> [w774 w776]
            tunnel: [w774 w775] -> w768
            frame False {
            }
            frame True {
              n299 = Not A Number/Path/Refnum?(number/path/refnum=w779) -> (NaN/Path/Refnum?=w780:bool)
              n300 = Not A Number/Path/Refnum?(number/path/refnum=w778) -> (NaN/Path/Refnum?=w782:bool)
              n301 = Exclusive Or(1:w782, 2:w780) -> (0:w781:bool)
              n302 = case shown="True" w781 {
                tunnel: w780 -> [_ w790]
                tunnel: w779 -> [_ w789]
                tunnel: w778 -> [_ w788]
                tunnel: w777 -> [_ w787]
                tunnel: w776 -> [w783 w786]
                tunnel: [w783 w785] -> w775
                frame False {
                }
                frame True {
                  n303 = Select(t=w788, s=w790, f=w789) -> (s? t:f=w784:dbl)
                  n304 = case shown="2" w787 {
                    tunnel: w786 -> [w793 w796 w799]
                    tunnel: [w792 w795 w798] -> w785
                    tunnel: w784 -> [w791 w794 w797]
                    frame 0, Default {
                      n305 = Bundle By Name(cluster=w793, "Start X"=w791, "End X"=w791) -> (w792:T1)
                    }
                    frame 1 {
                      n306 = Bundle By Name(cluster=w796, "Start Y"=w794, "End Y"=w794) -> (w795:T1)
                    }
                    frame 2 {
                      n307 = Bundle By Name(cluster=w799, "Start Z"=w797, "End Z"=w797) -> (w798:T1)
                    }
                  }
                }
              }
            }
          }
        }
      }
      frame "Check for position NaNs" {
        n308 = global read "Extra_Commands_Global.vi" "Skip Traverse Position Demand"() -> (w848:string)
        n309 = Unbundle By Name(w851) -> ("Extra Commands"=w847:string, "Start X"=w860:dbl, "Start Y"=w858:dbl, "Start Z"=w859:dbl, "End X"=w857:dbl, "End Y"=w856:dbl, "End Z"=w855:dbl)
        n310 = call "Extra_Commands.vi"("String to Search"=w847, "Command"=w848) -> ("Command Found"=w845:bool)  [unwired: 1 in, 4 out]
        n311 = case shown="False" w845 {
          tunnel: w860 -> [w875 _]
          tunnel: w859 -> [w874 _]
          tunnel: w858 -> [w873 _]
          tunnel: w857 -> [w872 _]
          tunnel: w856 -> [w871 _]
          tunnel: w855 -> [w870 _]
          tunnel: [w866 w876] -> w854
          tunnel: [w865 TRUE] -> w853
          tunnel: "" -> [w864 w876]
          frame False {
            n312 = Build Array(w875, w873, w874, w872, w871, w870) -> (w869:dbl[])
            n313 = Not A Number/Path/Refnum?(number/path/refnum=w869) -> (NaN/Path/Refnum?=w868:bool[])
            n314 = Or Array Elements(Boolean array=w868) -> (logical OR=w865:bool)
            n315 = Select(t="Some of the Start and End positions are NaN.\n" ("f"), s=w865, f=w864) -> (s? t:f=w866:string)
          }
          frame True {
          }
        }
        n316 = case shown="\"Set Tunnel Speed Only\", Default" w849 {
          tunnel: w853 -> [_ w882]
          tunnel: ["Check source details" ("t") w881] -> w852
          frame "Multi-Axis Profile" {
          }
          frame "Set Tunnel Speed Only", Default {
            n317 = Select(t="Check source details", s=w882, f="Check profile rows") -> (s? t:f=w881:string)
          }
        }
        n318 = Concatenate Strings(w862, w854) -> (w861:string)
      }
      frame "Check for Start NaNs" {
        n319 = Unbundle By Name(w888) -> ("Extra Commands"=w884:string, "Start X"=w893:dbl, "Start Y"=w891:dbl, "Start Z"=w892:dbl)
        n320 = global read "Extra_Commands_Global.vi" "Skip Traverse Position Demand"() -> (w885:string)
        n321 = call "Extra_Commands.vi"("String to Search"=w884, "Command"=w885) -> ("Command Found"=w883:bool)  [unwired: 1 in, 4 out]
        n322 = case shown="True" w883 {
          tunnel: w893 -> [w905 _]
          tunnel: w892 -> [w904 _]
          tunnel: w891 -> [w903 _]
          tunnel: "" -> [w900 w906]
          tunnel: [w898 w906] -> w889
          frame False {
            n323 = Build Array(w905, w903, w904) -> (w902:dbl[])
            n324 = Not A Number/Path/Refnum?(number/path/refnum=w902) -> (NaN/Path/Refnum?=w901:bool[])
            n325 = Or Array Elements(Boolean array=w901) -> (logical OR=w897:bool)
            n326 = Select(t="Some of the Start coordinates are NaN.\n" ("f"), s=w897, f=w900) -> (s? t:f=w898:string)
          }
          frame True {
          }
        }
        n327 = Concatenate Strings(w895, w889) -> (w894:string)
      }
      frame "Check profile rows" {
        n328 = call "Create_Pos_array.vi"("Traverse line"=w916) -> ("Traverse line Out"=w915:T1, "Error Messages"=w914:string)  [unwired: 7 out]
        n329 = Unbundle By Name(w916) -> ("Start X"=w938:dbl, "Start Y"=w937:dbl, "Start Z"=w936:dbl, "End X"=w935:dbl, "End Y"=w934:dbl, "End Z"=w933:dbl, "Specific Arguments"=w927:string, "Spacing"=w922:T2, "No. of pts."=w921:i32)
        n330 = local read "Fixed Axis"() -> (w920:bool[])
        n331 = Build Array(w938, w937, w936) -> (w918:dbl[])
        n332 = Build Array(w935, w934, w933) -> (w919:dbl[])
        n333 = case shown="\"Linear\"" w922 {
          tunnel: w927 -> [_ _ _ _ w973]
          tunnel: ["" w946 "\"N/A\" is not a valid point spacing.\n" "" w968] -> w926
          tunnel: w921 -> [_ _ _ _ w972]
          tunnel: w920 -> [_ w944 _ _ _]
          tunnel: w919 -> [_ w951 _ _ _]
          tunnel: w918 -> [_ w950 _ _ _]
          frame "Linear" {
          }
          frame "Log" {
            n334 = for {
              tunnel: w951 -> [w955] mode=indexing
              tunnel: w950 -> [w954] mode=indexing
              tunnel: [w953] -> w949 mode=indexing
              tunnel: w944 -> [w952] mode=indexing
              n335 = case shown="False" w952 {
                tunnel: w955 -> [w961 _]
                tunnel: w954 -> [w960 _]
                tunnel: [w956 FALSE] -> w953
                frame False {
                  w959 = 0.001 ("y")
                  n336 = Less?(x=w961, y=w959) -> (x < y?=w957:bool)
                  n337 = Less?(x=w960, y=w959) -> (x < y?=w958:bool)
                  n338 = Or(x=w957, y=w958) -> (x .or. y?=w956:bool)
                }
                frame True {
                }
              }
            }
            n339 = Or Array Elements(Boolean array=w949) -> (logical OR=w948:bool)
            n340 = Select(t="For log spacing, Start & End positions must be greater than 0.0001.", s=w948, f="") -> (s? t:f=w946:string)
          }
          frame "N/A" {
          }
          frame "Gauss" {
          }
          frame "Specified" {
            n341 = call "Get_array_values_fr_String.vi"("String Value"=w973) -> ("Numeric Array"=w967:dbl[])  [unwired: 1 out]
            n342 = Array Size(array=w967) -> (size(s)=w966:i32)
            n343 = Decrement(x=w966) -> (x-1=w965:i32)
            n344 = Equal?(x=w965, y=w972) -> (x = y?=w971:bool)
            n345 = Select(t="", s=w971, f="The No of points and No of Arguments do not match.\n") -> (s? t:f=w968:string)
          }
        }
        n346 = for {
          tunnel: w920 -> [w979] mode=indexing
          tunnel: w918 -> [w978] mode=indexing
          tunnel: w919 -> [w977] mode=indexing
          tunnel: [w976] -> w932 mode=indexing
          shift-right: [w974] -> w911
          shift-left: bool[] [] -> [w975]
          n347 = case shown="False" w979 {
            tunnel: w978 -> [w983 w989]
            tunnel: w977 -> [w984 w988]
            tunnel: [TRUE w987] -> w976
            tunnel: w975 -> [w981 w986]
            tunnel: [w980 w986] -> w974
            frame False {
              n348 = Not Equal?(x=w983, y=w984) -> (x != y?=w982:bool)
              n349 = Build Array (concatenate)(w981, w982) -> (w980:bool[])
            }
            frame True {
              n350 = Equal?(x=w989, y=w988) -> (x = y?=w987:bool)
            }
          }
        }
        n351 = Array Size(array=w911) -> (size(s)=w910:i32)
        n352 = And Array Elements(Boolean array=w932) -> (logical AND=w931:bool)
        n353 = Or Array Elements(Boolean array=w911) -> (logical OR=w908:bool)
        n354 = Not Equal To 0?(x=w910) -> (x != 0?=w909:bool)
        n355 = And(x=w908, y=w909) -> (x .and. y?=w907:bool)
        n356 = Select(t="", s=w931, f="This profile moves more than one axis.\n") -> (s? t:f=w928:string)
        n357 = Select(t="", s=w907, f="The start and end points are the same for this profile.\n") -> (s? t:f=w924:string)
        n358 = Concatenate Strings(w914, w924, w928, w926) -> (w941:string)
        n359 = Concatenate Strings(w940, w941) -> (w939:string)
      }
      frame "Check source details" {
        n360 = Unbundle By Name(w1001) -> ("Emission Rate (l/min)"=w1003:dbl, "Density Ratio"=w993:string)  [unwired: 1 out]
        n361 = Empty String/Path?(string/path=w993) -> (empty?=w994:bool)
        n362 = Equal?(x=w993, y="---------" ("f")) -> (x = y?=w992:bool)
        n363 = Or(x=w994, y=w992) -> (x .or. y?=w991:bool)
        n364 = Greater Than 0?(x=w1003) -> (x > 0?=w998:bool)
        n365 = And(x=w998, y=w991) -> (x .and. y?=w1002:bool)
        n366 = case shown="False" w1002 {
          tunnel: w1001 -> [w1006 w1009]
          tunnel: [w1006 w1007] -> w1000
          frame False {
          }
          frame True {
            (unwired) "The Density Ratio Box should contain either:\nCarrier 1 Only\nCarrier 2 Only\nor the relative density ratio of the mixed gas with respect to air" ("f")
            n367 = Bundle By Name(cluster=w1009, "Density Ratio"="Carrier 1 Only") -> (w1007:T1)
          }
        }
        n368 = Select(t="Check source detail 2", s=w998, f="check entered filename etc") -> (s? t:f=w996:string)
      }
      frame "Check source detail 2" {
        n369 = Unbundle By Name(w1033) -> ("Trace Gas Concentration (%)"=w1034:dbl, "Density Ratio"=w1035:string)
        n370 = To Upper Case(1:w1035) -> (0:w1018:string)
        n371 = To Upper Case(1:"Carrier 1 Only") -> (0:w1020:string)
        n372 = To Upper Case(1:"Carrier 2 Only") -> (0:w1019:string)
        n373 = In Range and Coerce(upper limit=ext 3.01 ("hi"), x=w1034, lower limit=ext 0.0 ("lo")) -> (In Range?=w1015:bool)  [unwired: 1 out]
        n374 = Equal?(x=w1018, y=w1020) -> (x = y?=w1025:bool)
        n375 = Equal?(x=w1018, y=w1019) -> (x = y?=w1024:bool)
        n376 = Fract/Exp String To Number(string=w1018) -> (number=w1026:dbl)  [unwired: 4 out]
        n377 = In Range and Coerce(upper limit=ext 10.0 ("hi"), x=w1026, lower limit=ext 0.05 ("lo")) -> (In Range?=w1023:bool)  [unwired: 1 out]
        n378 = Compound Arithmetic op=OR(w1025, w1024, w1023) -> (w1010:bool)
        n379 = Select(t="", s=w1015, f="The Trace Gas Concentration must be within the range of 0 to 3%.\n") -> (s? t:f=w1011:string)
        n380 = Select(t="", s=w1010, f="The Density Ratio Box should contain either:\nCarrier 1 Only\nCarrier 2 Only\nor the relative density ratio of the mixed gas with respect to air") -> (s? t:f=w1012:string)
        n381 = Concatenate Strings(w1011, w1012) -> (w1036:string)
        n382 = Concatenate Strings(w1038, w1036) -> (w1037:string)
      }
      frame "check entered filename etc" {
        n383 = local read "Checks"() -> (w1051:string[])
        n384 = for {
          tunnel: w1051 -> [w1058] mode=indexing
          tunnel: [w1063] -> w1052 mode=indexing
          tunnel: w1048 -> [w1062]
          shift-right: [w1060] -> w1042
          shift-left: w1043 -> [w1061]
          tunnel: [w1059] -> w1041 mode=indexing
          n385 = case shown="\"Number:Of:Points\"" w1058 {
            tunnel: w1061 -> [w1065 w1073 w1095 w1110]
            tunnel: [w1066 w1076 w1101 w1106] -> w1063
            tunnel: w1062 -> [_ _ w1104 _]
            tunnel: [w1065 w1073 w1093 w1110] -> w1060
            tunnel: [TRUE ("cancelled") TRUE ("cancelled") w1088 TRUE ("cancelled")] -> w1059
            tunnel: w1058 -> [_ _ _ w1108]
            frame "Number:Of:Points" {
              n386 = Unbundle By Name(w1065) -> ("No. of pts."=w1068:i32)
              n387 = Greater?(x=w1068, y=1) -> (0:w1070:bool)
              n388 = Select(t="", s=w1070, f="For a profile the number of points should be more than 1.\n" ("Format String")) -> (s? t:f=w1066:string)
            }
            frame "Averaging:Time:(mins)" {
              n389 = Unbundle By Name(w1073) -> ("Averaging time (min)"=w1075:dbl)
              n390 = Greater Than 0?(x=w1075) -> (x > 0?=w1074:bool)
              n391 = Select(t="", s=w1074, f="The averaging time should be greater than zero.\n" ("Format String")) -> (s? t:f=w1076:string)
            }
            frame "Filename:HD:Users" {
              w1102 = FALSE  # Show Error handler
              n392 = Unbundle By Name(w1095) -> ("Filename"=w1079:path, "Row No"=w1090:i32, "Row Type Selector"=w1086:T3)
              n393 = call "Row_type_selector_string.vi"("Mode"=w1086) -> ("Output string"=w1085:string)
              n394 = call "Current_Filepath.vi"("Filename in"=w1079, "Data Type"="Results") -> ("Filename Out"=w1080:path)  [unwired: 1 out]
              n395 = Path To String(path=w1080) -> (string=w1099:string)
              n396 = Not A Number/Path/Refnum?(number/path/refnum=w1080) -> (NaN/Path/Refnum?=w1083:bool)
              n397 = Equal?(x=Multi_run_mode."Run VI Named:" ("Mode"), y=w1104) -> (x = y?=w1103:bool)
              n398 = Match Pattern(string=w1099, regular expression="-------" ("f")) -> (match substring=w1098:string)  [unwired: 4 out]
              n399 = Empty String/Path?(string/path=w1098) -> (empty?=w1084:bool)
              n400 = Format Into String(format string=" For Row  %d %s." ("Comment"), w1090, w1085) -> (resulting string=w1089:string)  [unwired: 2 in, 1 out]
              n401 = Compound Arithmetic op=AND(w1084, invert w1083) -> (w1082:bool)
              n402 = Select(t=w1080, s=w1082, f=path "") -> (s? t:f=w1097:path)
              n403 = call "Results_filename_checker.vi"("Filelength"=35, "Warn if Already Exists"=w1103, "Comment"=w1089, "Show Error handler"=w1102, "Results file"=w1097) -> ("Error String"=w1101:string, "cancelled"=w1092:bool, "Results file output"=w1094:path)  [unwired: 1 out]
              n404 = Bundle By Name(cluster=w1095, "Filename"=w1094) -> (w1093:T1)
              n405 = Not(x=w1092) -> (.not. x?=w1088:bool)
            }
            frame "No Match", Default {
              n406 = Concatenate Strings(w1108, " Has not been programmed.\n" ("string")) -> (w1106:string)
            }
          }
        }
        n407 = local read "Editted Row"() -> (w1045:bool)
        n408 = And Array Elements(Boolean array=w1041) -> (logical AND=w1040:bool)
        n409 = Concatenate Strings(w1052) -> (w1050:string)
        n410 = Concatenate Strings(w1049, w1050) -> (w1044:string)
        n411 = Empty String/Path?(string/path=w1044) -> (empty?=w1047:bool)
        n412 = case shown="False" w1047 {
          tunnel: ["Open Front Panel" w1056] -> w1046
          tunnel: w1045 -> [_ w1057]
          frame False {
          }
          frame True {
            n413 = Select(t="Close Front Panel", s=w1057, f="End") -> (s? t:f=w1056:string)
          }
        }
      }
      frame "Open Front Panel" {
        w1115 = TRUE  # Front Panel Window:Open
        n414 = Current VI's Path() -> (path=w1116:path)
        n415 = call "Open_Close_Front_Panel.ph.vi"("Front Panel Window:Open"=w1115, "VI path"=w1116) -> ()  [unwired: 2 out]
        n416 = local write "Editted Row"(TRUE ("Editted Row")) -> ()
        n417 = local write "Execution Row"(w1112) -> ()
      }
      frame "What to do next?" {
        w1126 = ""
        w1124 = "[\r\n]"
        n418 = local read "Execution Row"() -> (w1122:T1)
        n419 = Wait Until Next ms Multiple(millisecond multiple=u32 100) -> ()  [unwired: 1 out]
        n420 = Unbundle By Name(w1122) -> ("Row Type Selector"=w1138:T3, "Specific Arguments"=w1133:string, "Extra Commands"=w1131:string, "Density Ratio"=w1125:string)
        n421 = Not Equal?(x=Multi_run_mode."Blank Row" ("Mode"), y=w1138) -> (x != y?=w1134:bool)
        n422 = call "Replace_Character.vi"("Replace with"=w1126, "Input String"=w1133, "Search For"=w1124) -> ("Output string"=w1132:string)  [unwired: 1 out]
        n423 = call "Replace_Character.vi"("Replace with"=w1126, "Input String"=w1131, "Search For"=w1124) -> ("Output string"=w1130:string)  [unwired: 1 out]
        n424 = call "Replace_Character.vi"("Replace with"=w1126, "Input String"=w1125, "Search For"=w1124) -> ("Output string"=w1123:string)  [unwired: 1 out]
        n425 = Compound Arithmetic op=OR("Edit in Excel", "OK") -> (w1135:bool)
        n426 = Bundle By Name(cluster=w1122, "Specific Arguments"=w1132, "Extra Commands"=w1130, "Density Ratio"=w1123) -> (w1120:T1)
        n427 = Compound Arithmetic op=AND(w1135, w1134) -> (w1128:bool)
        n428 = Not Equal?(x=w1120, y=w1122) -> (x != y?=w1121:bool)
        n429 = Not(x="Edit in Excel") -> (.not. x?=w1119:bool)
        n430 = case shown="True" w1121 {
          tunnel: w1120 -> [_ w1142]
          frame False {
          }
          frame True {
            n431 = local write "Execution Row"(w1142) -> ()
          }
        }
        n432 = case shown="True" w1119 {
          tunnel: ["Close Front Panel" w1147] -> w1127
          tunnel: w1128 -> [_ w1146]
          frame False {
          }
          frame True {
            n433 = Select(t="Clean Up Row", s=w1146, f="What to do next?") -> (s? t:f=w1147:string)
          }
        }
        "Error Comments" <- w1129
      }
      frame "Clean Up Row" {
        n434 = call "Traverse_Control_Ch_Names.vi"("Mode"=T4."All Channel Names") -> ("Channel names"=w1156:string[])  [unwired: 1 in]
        n435 = call "Trav_Cluster_to_Row.vi"("Traverse line in"=w1151, "Row Number"=w1152, "Channel names"=w1156) -> ("Traverse line Out"=w1154:T1)  [unwired: 4 out]
      }
      frame "Close Front Panel" {
        w1160 = FALSE  # Front Panel Window:Open
        n436 = Current VI's Path() -> (path=w1161:path)
        n437 = call "Open_Close_Front_Panel.ph.vi"("Front Panel Window:Open"=w1160, "VI path"=w1161) -> ()  [unwired: 2 out]
      }
      frame "End" {
        n438 = local read "Editted Row"() -> (w1169:bool)
        n439 = case shown="True" w1169 {
          tunnel: w1168 -> [w1172 w1175]
          tunnel: [w1172 w1174] -> w1166
          tunnel: w1167 -> [_ w1173]
          frame False {
          }
          frame True {
            n440 = call "Traverse_Control_Ch_Names.vi"("Mode"=T4."All Channel Names") -> ("Channel names"=w1176:string[])  [unwired: 1 in]
            n441 = call "Trav_Cluster_to_Row.vi"("Traverse line in"=w1175, "Row Number"=w1173, "Channel names"=w1176) -> ("Traverse line Out"=w1174:T1)  [unwired: 4 out]
          }
        }
        n442 = local write "Error Comments"(w1170) -> ()
      }
    }
    "Traverse line Out" <- w8
  }
  "Execution Row Out" <- w2
  "Continue?" <- w1
